vi "LA_data_decode.vi"(10 "Data In":u8[](array[numeric]), 11 "N":dbl) -> (1 "Byte Time Stamp":dbl[](array[numeric]), 2 "Index Array":u8[](array[numeric]), 3 "Data Out":u8[](array[numeric]))   [LabVIEW 2012]
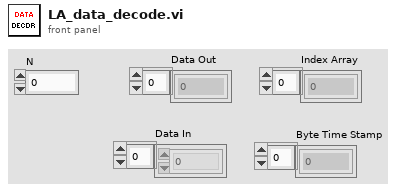
[diagram p1: front panel]
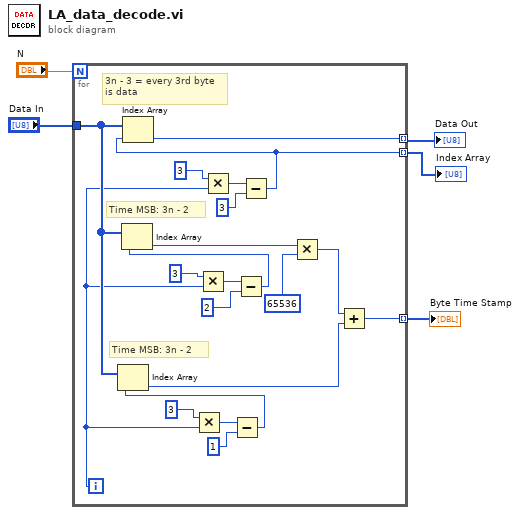
[diagram p0: block diagram]
diagram:
  n1 = for {
    N: "N" -> [_]
    tunnel: [w21] -> w2 mode=indexing
    tunnel: [w23] -> w4 mode=indexing
    tunnel: "Data In" -> [w12]
    tunnel: [w6] -> w1 mode=indexing
    i -> [w11]
    # "Time MSB: 3n - 2"
    # "Time MSB: 3n - 2"
    # "3n - 3 = every 3rd byte \nis data"
    n2 = Multiply(x=3, y=w11) -> (x*y=w15:i32)
    n3 = Multiply(x=3, y=w11) -> (x*y=w19:i32)
    n4 = Multiply(x=3, y=w11) -> (x*y=w24:i32)
    n5 = Subtract(x=w15, y=1) -> (x-y=w13:i32)
    n6 = Index Array(array=w12, index=w13) -> (element=w7:u8)
    n7 = Subtract(x=w19, y=2) -> (x-y=w17:i32)
    n8 = Index Array(array=w12, index=w17) -> (element=w10:u8)
    n9 = Subtract(x=w24, y=3) -> (x-y=w21:i32)
    n10 = Index Array(array=w12, index=w21) -> (element=w23:u8)
    n11 = Multiply(x=w10, y=65536) -> (x*y=w8:i32)
    n12 = Add(x=w8, y=w7) -> (x+y=w6:i32)
  }
  "Data Out" <- w4
  "Index Array" <- w2
  "Byte Time Stamp" <- w1
